vi "Strain Gauge Reading continuous.vi"() -> ()   [LabVIEW 2022 SP3]
panel:
  out "Waveform Chart 2":dynamicdata(graph)
  out "Waveform Chart":dynamicdata(graph)
  in  "stop (F)":bool
  out "Saving Data":bool
  out "Filename Out":path
  in  "Filename":path=path "StrainGaugeTest/test.xlsx"
  in  "Enable":bool=TRUE
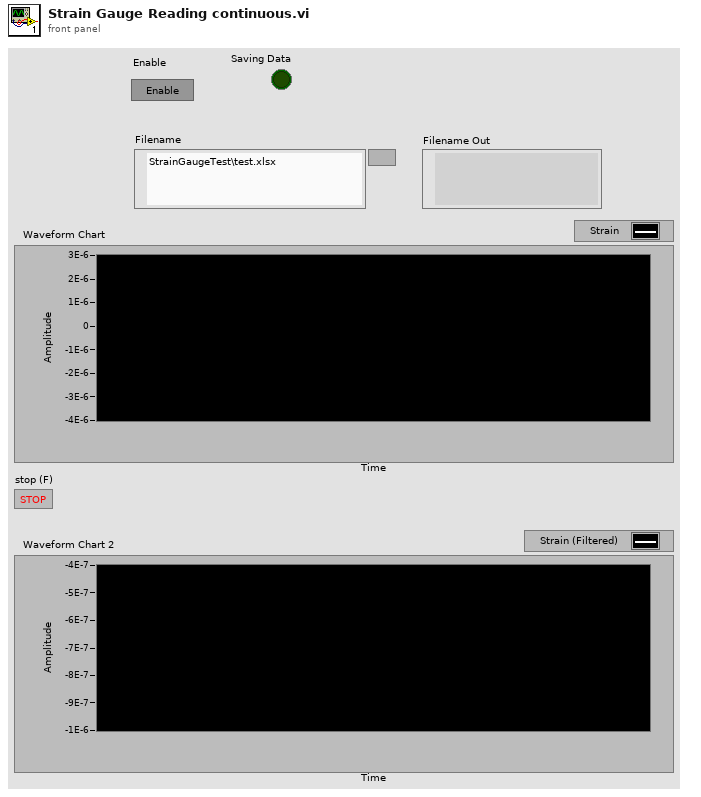
[diagram p1: front panel]
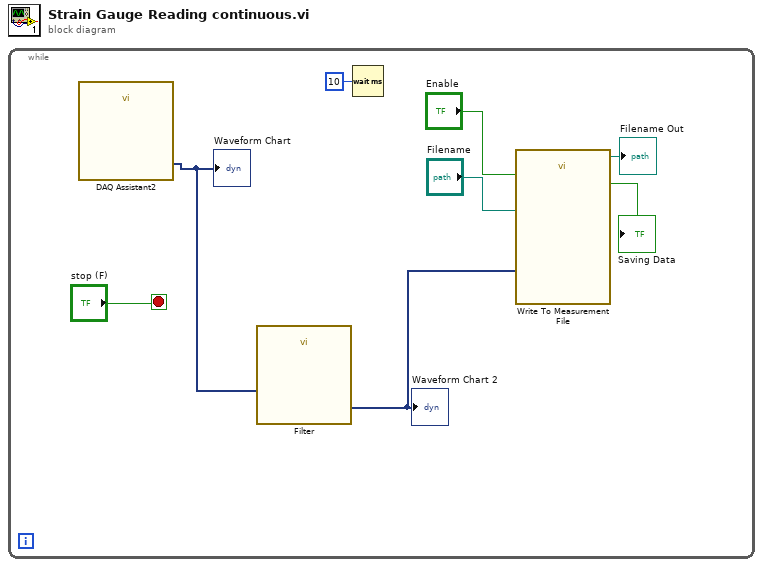
[diagram p0: block diagram]
diagram:
  n1 = while {
    stop <- "stop (F)" stop-if-true
    n2 = call "DAQ Assistant2"() -> ("data"=w2:dynamicdata)  [unwired: 16 in, 3 out]
    "Waveform Chart" <- w2
    n3 = call "Filter"("Signal"=w2) -> ("Filtered Signal"=w1:dynamicdata)  [unwired: 9 in, 1 out]
    "Waveform Chart 2" <- w1
    n4 = Wait (ms)(milliseconds to wait=u32 10) -> ()  [unwired: 1 out]
    n5 = call "Write To Measurement File"("Signals"=w1, "Enable"="Enable", "Filename"="Filename") -> ("Filename Out"=→"Filename Out":path, "Saving Data"=→"Saving Data":bool)  [unwired: 14 in, 1 out]
  }
